vi "m1m3_waitForCompletion_TranslateM1M3.vi"(8 "error in (no error)":errorcluster, 11 "waitComplete_Ctl":cluster{"cmdSeqNum":i32, "timeout":u32}) -> (0 "error out":errorcluster, 2 "function return":i32, 3 "waitComplete_Ctl out":cluster{"cmdSeqNum":i32, "timeout":u32})   [LabVIEW 2016, in "SALLV_m1m3.lvlib"]
doc: "int m1m3_shm_waitForCompletion_TranslateM1M3LV(m1m3_waitCompleteLV *waitComplete_Ctl);"
uses:
  SALLV_m1m3.lvlib
  SALLV_m1m3.so
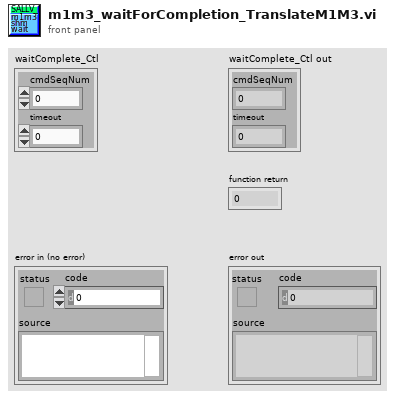
[diagram p1: front panel]
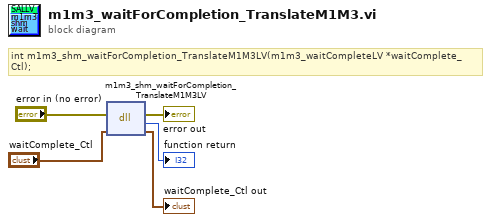
[diagram p0: block diagram]
diagram:
  # "int m1m3_shm_waitForCompletion_TranslateM1M3LV(m1m3_waitCompleteLV *waitComplete_Ctl);"
  n1 = dll-call lib="opt/CODE/SALLV_m1m3/SALLV_m1m3.*" fn="m1m3_shm_waitForCompletion_TranslateM1M3LV"(error in="error in (no error)", "waitComplete_Ctl"="waitComplete_Ctl") -> (error out=→"error out":errorcluster, →"function return":i32, "waitComplete_Ctl"=→"waitComplete_Ctl out":cluster{"cmdSeqNum":i32, "timeout":u32})  [unwired: 2 in, 1 out]
